vi "TurnFGV.vi"(10 "Énum":enum16{"set", "get"}(ring)=enum."get", 11 "set":bool) -> (3 "get":bool)   [LabVIEW 2020]
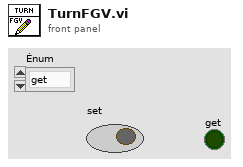
[diagram p1: front panel]
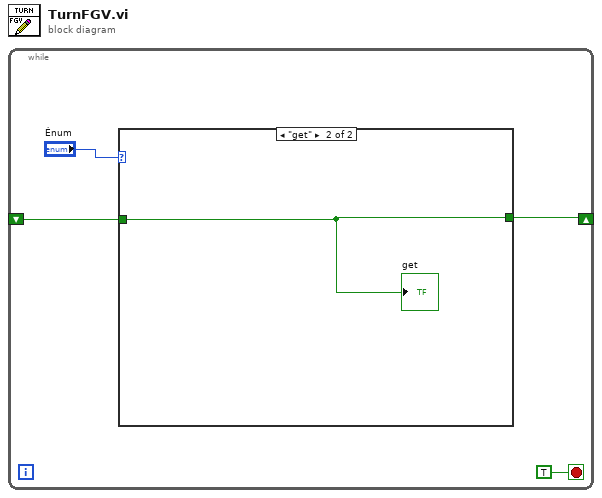
[diagram p0: block diagram]
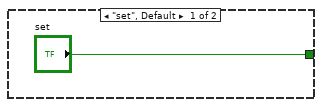
[diagram p2: hidden frame]
diagram:
  n1 = while {
    shift-right: [w2] -> _
    shift-left: _ -> [w1]
    stop <- TRUE stop-if-true
    n2 = case shown="\"get\"" "Énum" {
      tunnel: ["set" w6] -> w2
      tunnel: w1 -> [_ w6]
      frame "set", Default {
      }
      frame "get" {
        "get" <- w6
      }
    }
  }
